vi "Vision Tracking 1.vi"(0 "Image In":T2, 1 "Red or Hue Range (Color Threshold 1)":cluster{"Lower value":i32, "Upper value":i32}={"Lower value"=97, "Upper value"=153}, 2 "Green or Sat Range (Color Threshold 1)":cluster{"Lower value":i32, "Upper value":i32}={"Lower value"=0, "Upper value"=196}, 3 "Blue or Luma or Val or Inten Range (Color Threshold 1)":cluster{"Lower value":i32, "Upper value":i32}={"Lower value"=40, "Upper value"=151}, 7 "error in":errorcluster) -> (20 "Image Out":T2, 21 "Matches (Geometric Matching 1)":T1[](array[typedef]) {"Correlation Score" format="%.2f"; "Target Template Curve Score" format="%.2f"; "Template Target Curve Score" format="%.2f"; "Bounding Box"."y" format="%.2f"; "Bounding Box"."x" format="%.2f"; "Position"."y" format="%.2f"; "Position"."x" format="%.2f"; "Score" format="%.2f"; "Scale" format="%.2f"; "Angle" format="%.2f"; "Occlusion %" format="%.2f"}, 22 "Calibrated Matches (Geometric Matching 1)":T1[](array[typedef]) {"Correlation Score" format="%.2f"; "Target Template Curve Score" format="%.2f"; "Template Target Curve Score" format="%.2f"; "Bounding Box"."y" format="%.2f"; "Bounding Box"."x" format="%.2f"; "Position"."y" format="%.2f"; "Position"."x" format="%.2f"; "Score" format="%.2f"; "Scale" format="%.2f"; "Angle" format="%.2f"; "Occlusion %" format="%.2f"}, 23 "Number of Matches (Geometric Matching 1)":i32, 27 "error out":errorcluster)   [LabVIEW 2015]
uses:
  <vilib>/vision/Image Controls.llb/IMAQ Image.ctl
  <vilib>/vision/Pattern Matching.llb/IMAQ GM Match Report.ctl
  <vilib>/vision/Pattern Matching.llb/IMAQ Curve Parameters.ctl
  <vilib>/vision/Pattern Matching.llb/IMAQ Match Range Setting.ctl
  <vilib>/vision/NI_Vision_Development_Module.lvlib
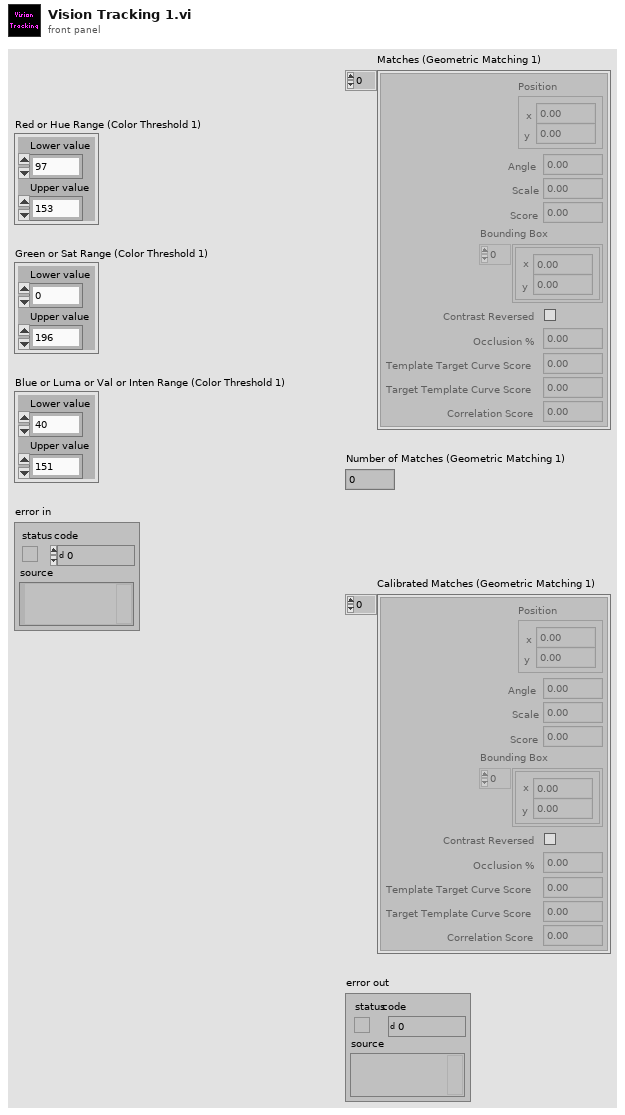
[diagram p1: front panel]
types:
  T1 = typedef "IMAQ GM Match Report.ctl" = cluster{"Position":cluster{"x":sgl, "y":sgl}, "Angle":sgl, "Scale":sgl, "Score":sgl, "Bounding Box":cluster{"x":sgl, "y":sgl}[], "Contrast Reversed":bool, "Occlusion %":sgl, "Template Target Curve Score":sgl, "Target Template Curve Score":sgl, "Correlation Score":sgl}
  T2 = typedef "IMAQ Image.ctl" = refnum<image>
  T3 = typedef "IMAQ Curve Parameters.ctl" = cluster{"Extraction Mode":u32, "Edge Threshold":i32, "Edge Filter Size":u32, "Min Length":i32, "Row Search Step Size":i32, "Col Search Step Size":i32, "Max Endpoint Gap":i32, "Closed":bool, "Subpixel":bool}
  T4 = typedef "IMAQ Match Range Setting.ctl" = cluster{"Match Constraints":u32, "Min":dbl, "Max":dbl}
  T5 = cluster{"Curve Parameters":T3, "Match Mode":cluster{"Rotation":bool, "Scale":bool, "Occlusion":bool, "Reserved":bool, "Reserved":bool, "Reserved":bool}, "Range Settings":T4[], "Number of Matches":i32, "Minimum Match Score":sgl, "SubPixel Accuracy":bool, "Adv. Geometric Match Options 2":cluster{"Setup Data Item":u16, "Item Value":dbl}[]}
  T6 = cluster{"Global Rectangle":i32[], "Contours":cluster{"ID":enum32{"External", "Internal"}, "Type":u32, "Coordinates":i32[]}[]}
  T7 = enum32{"AutoM", "Close", "Dilate", "Erode", "Gradient", "Gradient in", "Gradient out", "HitMiss", "Open", "PClose", "POpen", "Thick", "Thin"}
  T8 = cluster{"histogram":u32[], "Minimal Value":sgl, "Maximal Value":sgl, "Starting Value":sgl, "Interval Width":sgl, "Mean Value":sgl, "Standard  Variation":sgl, "Area (pixels)":i32}
  T9 = typedef "Image Type" = u32
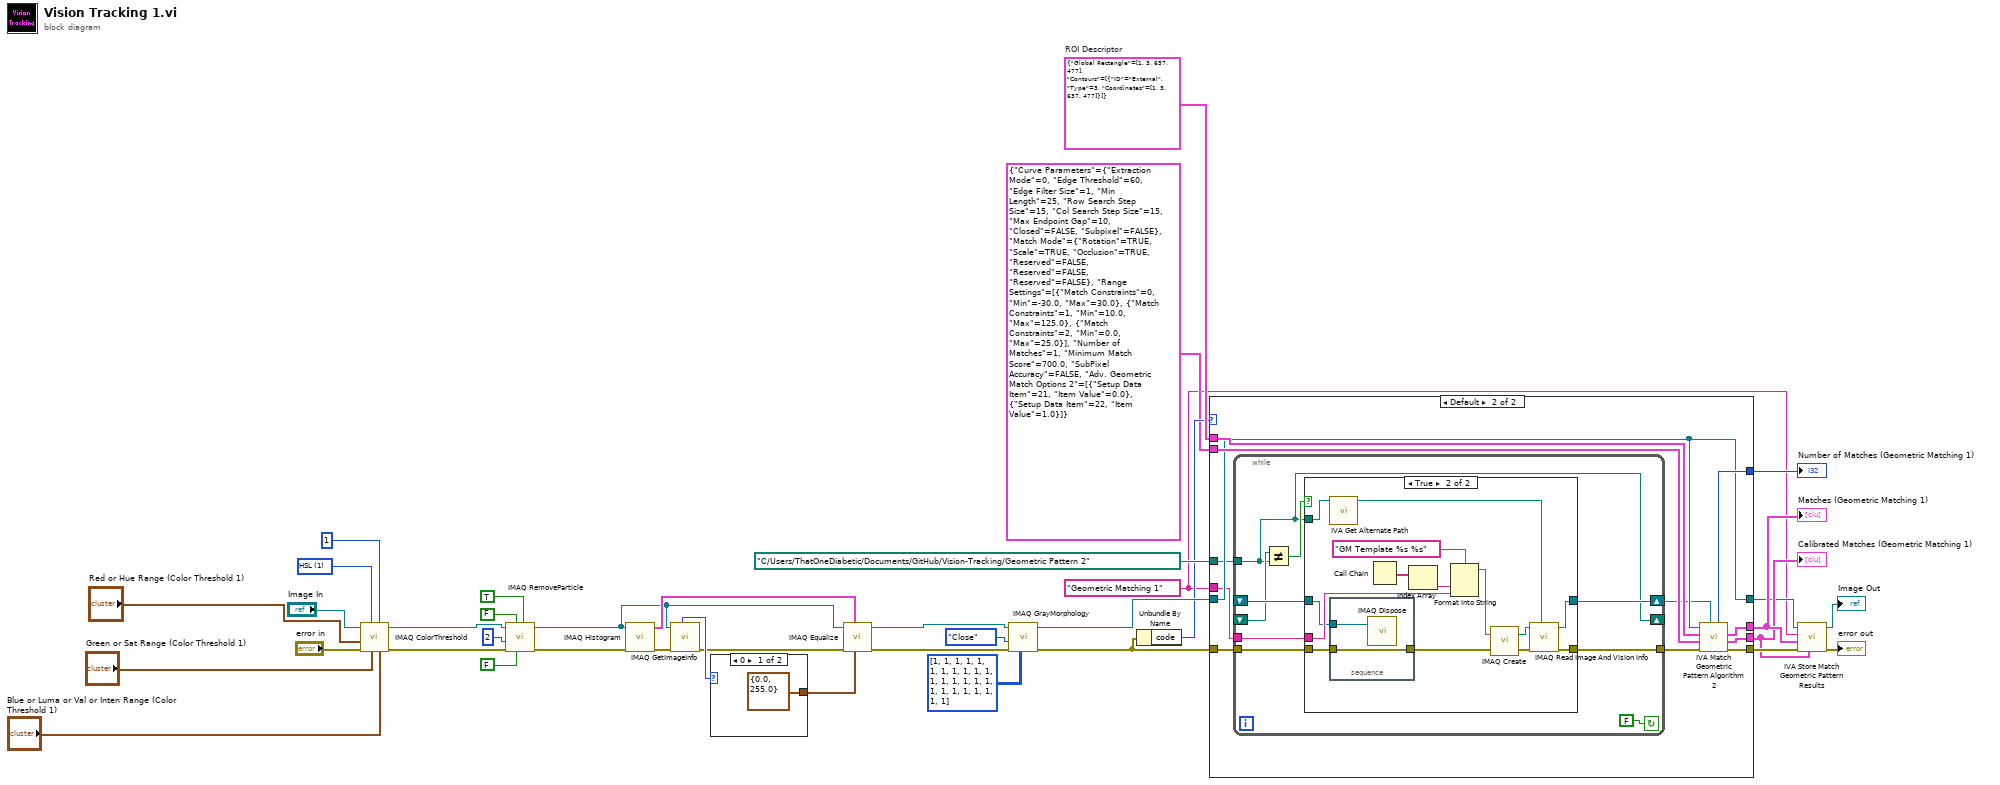
[diagram p0: block diagram]
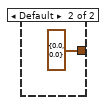
[diagram p4: hidden frame]
diagram:
  w1 = "Geometric Matching 1" ("Step Name")
  w13 = T6 {"Global Rectangle"=[1, 3, 637, 477], "Contours"=[{"ID"=enum."External", "Type"=3, "Coordinates"=[1, 3, 637, 477]}]}  # ROI Descriptor
  w37 = u16 1 items=["RGB", "HSL", "HSV", "HSI"] ("Color Mode")
  n1 = call "IMAQ ColorThreshold"("Blue or Luma or Val or Inten Range"="Blue or Luma or Val or Inten Range (Color Threshold 1)", "Replace Value"=1, "Green or Sat Range"="Green or Sat Range (Color Threshold 1)", "Color Mode"=w37, "error in (no error)"="error in", "Red or Hue Range"="Red or Hue Range (Color Threshold 1)", "Image Src"="Image In") -> ("error out"=w26:errorcluster, "Image Dst Out"=w27:T2)  [unwired: 1 in, 2 out]
  n2 = call "IMAQ RemoveParticle"("Connectivity 4/8 (8)"=TRUE, "Low Pass/High Pass (Low)"=FALSE, "Square/Hexa (Square)"=FALSE, "error in (no error)"=w26, "Number of Erosion"=2, "Image Src"=w27) -> ("error out"=w24:errorcluster, "Image Dst Out"=w22:T2)  [unwired: 1 in, 3 out]
  n3 = call "IMAQ Histogram"("error in (no error)"=w24, "Image"=w22) -> ("error out"=w21:errorcluster, "Histogram Report"=w25:T8)  [unwired: 3 in, 5 out]
  n4 = call "IMAQ GetImageInfo"("error in (no error)"=w21, "Image"=w22) -> ("error out"=w20:errorcluster, "Image Type"=w23:T9)  [unwired: 8 out]
  n5 = case shown="0" w23 {
    tunnel: [cluster{"Minimum":sgl, "Maximum":sgl} {"Minimum"=0.0, "Maximum"=255.0} ("Range") cluster{"Minimum":sgl, "Maximum":sgl} {"Minimum"=0.0, "Maximum"=0.0} ("Range")] -> w19
    frame 0 {
    }
    frame Default {
    }
  }
  n6 = call "IMAQ Equalize"("Range"=w19, "Histogram Report"=w25, "error in (no error)"=w20, "Image Src"=w22) -> ("error out"=w15:errorcluster, "Image Dst Out"=w16:T2)  [unwired: 2 in, 4 out]
  n7 = call "IMAQ GrayMorphology"("Structuring Element"=i32[][] [[1, 1, 1, 1, 1], [1, 1, 1, 1, 1], [1, 1, 1, 1, 1], [1, 1, 1, 1, 1], [1, 1, 1, 1, 1]], "error in (no error)"=w15, "Operation"=T7."Close", "Image Src"=w16) -> ("error out"=w5:errorcluster, "Image Dst Out"=w12:T2)  [unwired: 3 in, 3 out]
  n8 = Unbundle By Name(w5) -> ("code"=w4:i32)
  n9 = case shown="Default" w4 {
    tunnel: path "C:/Users/ThatOneDiabetic/Documents/GitHub/Vision-Tracking/Geometric Pattern 2" ("Template File Path") -> [_ w46]
    tunnel: w5 -> [_ w45]
    tunnel: T5 {"Curve Parameters"={"Extraction Mode"=0, "Edge Threshold"=60, "Edge Filter Size"=1, "Min Length"=25, "Row Search Step Size"=15, "Col Search Step Size"=15, "Max Endpoint Gap"=10, "Closed"=FALSE, "Subpixel"=FALSE}, "Match Mode"={"Rotation"=TRUE, "Scale"=TRUE, "Occlusion"=TRUE, "Reserved"=FALSE, "Reserved"=FALSE, "Reserved"=FALSE}, "Range Settings"=[{"Match Constraints"=0, "Min"=-30.0, "Max"=30.0}, {"Match Constraints"=1, "Min"=10.0, "Max"=125.0}, {"Match Constraints"=2, "Min"=0.0, "Max"=25.0}], "Number of Matches"=1, "Minimum Match Score"=700.0, "SubPixel Accuracy"=FALSE, "Adv. Geometric Match Options 2"=[{"Setup Data Item"=21, "Item Value"=0.0}, {"Setup Data Item"=22, "Item Value"=1.0}]} ("Settings") -> [_ w53]
    tunnel: w13 -> [_ w52]
    tunnel: w12 -> [w41 w47]
    tunnel: [_ w51] -> w10
    tunnel: [_ w50] -> w8
    tunnel: [_ w49] -> w7
    tunnel: [_ w48] -> w6
    tunnel: [w41 w47] -> w3
    tunnel: w1 -> [_ w42]
    frame -1074396199, -1074396198 {
      # "Discard Coordinate System Error"
    }
    frame Default {
      n10 = while {
        shift-right: [w62] -> w43
        shift-left: _ -> [w61]
        tunnel: [w59] -> w44
        tunnel: w45 -> [w58]
        tunnel: w46 -> [w54]
        tunnel: w42 -> [w57]
        shift-right: [w54] -> _
        shift-left: _ -> [w56]
        stop <- FALSE continue-if-true
        n11 = Not Equal?(x=w56, y=w54) -> (x != y?=w55:bool)
        n12 = case shown="True" w55 {
          tunnel: [w64 w76] -> w62
          tunnel: w61 -> [w64 w68]
          tunnel: [w63 w73] -> w59
          tunnel: w58 -> [w63 w69]
          tunnel: w57 -> [_ w70]
          tunnel: w54 -> [_ w66]
          frame False {
          }
          frame True {
            n13 = call <vilib>:"IVA Get Alternate Path.vi"("Path In"=w66) -> ("Path Out"=w65:path)  [unwired: 10 out]
            n14 = stacked-sequence {
              tunnel: w69 -> [w80]
              tunnel: w68 -> [w79]
              tunnel: [w80] -> w67
              frame #0 {
                n15 = call "IMAQ Dispose"("Image"=w79) -> ()  [unwired: 2 in, 4 out]
              }
            }
            n16 = Call Chain() -> (call chain=w72:string[])
            n17 = Index Array(array=w72) -> (element=w71:string)  [unwired: 1 in]
            n18 = Format Into String(format string="GM Template %s %s" ("Image Name"), w71, w70) -> (resulting string=w78:string)  [unwired: 2 in, 1 out]
            n19 = call "IMAQ Create"("Image Name"=w78, "error in (no error)"=w67) -> ("New Image"=w75:T2, "error out"=w74:errorcluster)  [unwired: 2 in, 1 out]
            n20 = call "IMAQ Read Image And Vision Info"("File Path"=w65, "error in (no error)"=w74, "Image"=w75) -> ("error out"=w73:errorcluster, "Image Out"=w76:T2)  [unwired: 1 in, 6 out]
          }
        }
      }
      n21 = call <vilib>:"IVA Match Geometric Pattern Algorithm 2.vi"("Template"=w43, "error in (no error)"=w44, "Settings"=w53, "ROI Descriptor"=w52, "Image"=w47) -> ("error out"=w51:errorcluster, "Calibrated Matches"=w49:T1[], "Matches"=w50:T1[], "Number of Matches"=w48:i32)  [unwired: 1 in, 2 out]
    }
  }
  "Matches (Geometric Matching 1)" <- w8
  "Number of Matches (Geometric Matching 1)" <- w6
  "Calibrated Matches (Geometric Matching 1)" <- w7
  n22 = call <vilib>:"IVA Store Match Geometric Pattern Results.vi"("Calibrated Matches"=w7, "error in (no error)"=w10, "Matches"=w8, "Step Name"=w1, "Image in"=w3) -> ("error out"=→"error out":errorcluster, "Image dup"=→"Image Out":T2)  [unwired: 5 out]
